vi "Timing 5min after 5min before.vi"() -> (1 "Mid Hour":bool)   [LabVIEW 2011]
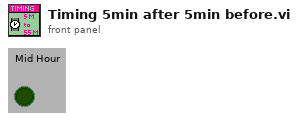
[diagram p1: front panel]
types:
  T1 = typedef "LVDateTimeRec.ctl" = cluster{"fractional second":dbl, "second":i32, "minute":i32, "hour":i32, "day of month":i32, "month":i32, "year":i32, "day of week":i32, "day of year":i32, "DST":i32}
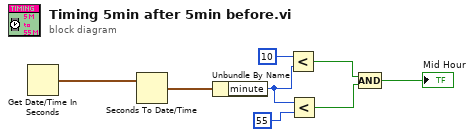
[diagram p0: block diagram]
diagram:
  n1 = Get Date/Time In Seconds() -> (seconds since 1Jan1904=w7:timestamp)
  n2 = Seconds To Date/Time(time stamp (now)=w7) -> (date time rec=w8:T1)  [unwired: 1 in]
  n3 = Unbundle By Name(w8) -> ("minute"=w6:i32)
  n4 = Less?(x=10, y=w6) -> (x < y?=w3:bool)
  n5 = Less?(x=w6, y=55) -> (x < y?=w2:bool)
  n6 = Compound Arithmetic op=AND(w3, w2) -> (→"Mid Hour":bool)
